vi "Write Pin.vi"(0 "Simulada in":refnum<class "Simulada.lvclass">, 5 "VISA resource name":refnum<visa-resource-name>, 7 "Pin":u16, 9 "Port 3":u16, 11 "error in (no error)":errorcluster, 12 "Set Pin":bool) -> (4 "Simulada out":refnum<class "Simulada.lvclass">, 6 "VISA resource name 2":refnum<visa-resource-name>, 15 "error out":errorcluster)   [LabVIEW 2020, in "Simulada.lvclass"]
uses:
  Simulada.lvclass
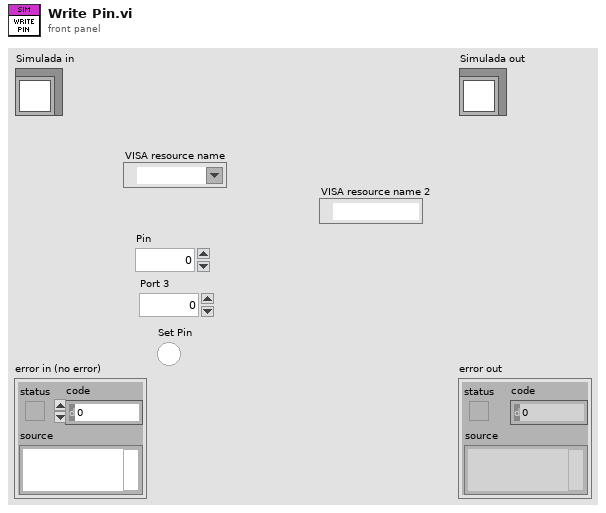
[diagram p1: front panel]
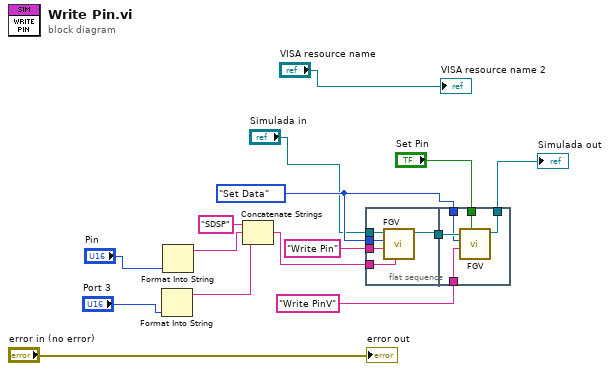
[diagram p0: block diagram]
diagram:
  w8 = enum16{"Get Data", "Set Data"}."Set Data" ("Enum")
  n1 = Format Into String("Port 3") -> (resulting string=w10:string)  [unwired: 3 in, 1 out]
  n2 = Format Into String("Pin") -> (resulting string=w11:string)  [unwired: 3 in, 1 out]
  n3 = Concatenate Strings("SDSP" ("string"), w11, w10) -> (w9:string)
  n4 = flat-sequence {
    tunnel: "Simulada in" -> [w20]
    tunnel: w8 -> [w18]
    tunnel: "Write Pin" ("Name") -> [w17]
    tunnel: w9 -> [w16]
    tunnel: [w19] -> w14
    tunnel: w14 -> [w25]
    tunnel: [w24] -> w4
    tunnel: "Set Pin" -> [w23]
    tunnel: w8 -> [w22]
    tunnel: "Write PinV" ("Name") -> [w21]
    frame #0 {
      n5 = call-dynamic "FGV.vi"("Simulada in"=w20, "Enum"=w18, "Name"=w17, "Data 2"=w16) -> ("Simulada out"=w19:refnum<class "Simulada.lvclass">)  [unwired: 4 in, 2 out]
    }
    frame #1 {
      n6 = call-dynamic "FGV.vi"("Simulada in"=w25, "Enum"=w22, "Name"=w21, "Data 2"=w23) -> ("Simulada out"=w24:refnum<class "Simulada.lvclass">)  [unwired: 4 in, 2 out]
    }
  }
  "error out" <- "error in (no error)"
  "Simulada out" <- w4
  "VISA resource name 2" <- "VISA resource name"
